vi "sub3.vi"(11 "Terminal in":refnum<vi>) -> (3 "Argument":T1)   [LabVIEW 2020, in "CSM-Helper.lvclass"]
uses:
  CSM-Helper.lvclass
  Typedef/Def-Argument Info.ctl
  <userlib>/_NEVSTOP/Communicable State Machine(CSM)/Communicable State Machine.lvlib
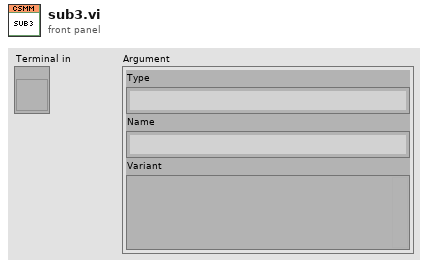
[diagram p1: front panel]
types:
  T1 = typedef "CSM-Helper.lvclass/Def-Argument Info.ctl" = cluster{"Type":string, "Name":string, "Variant":variant}
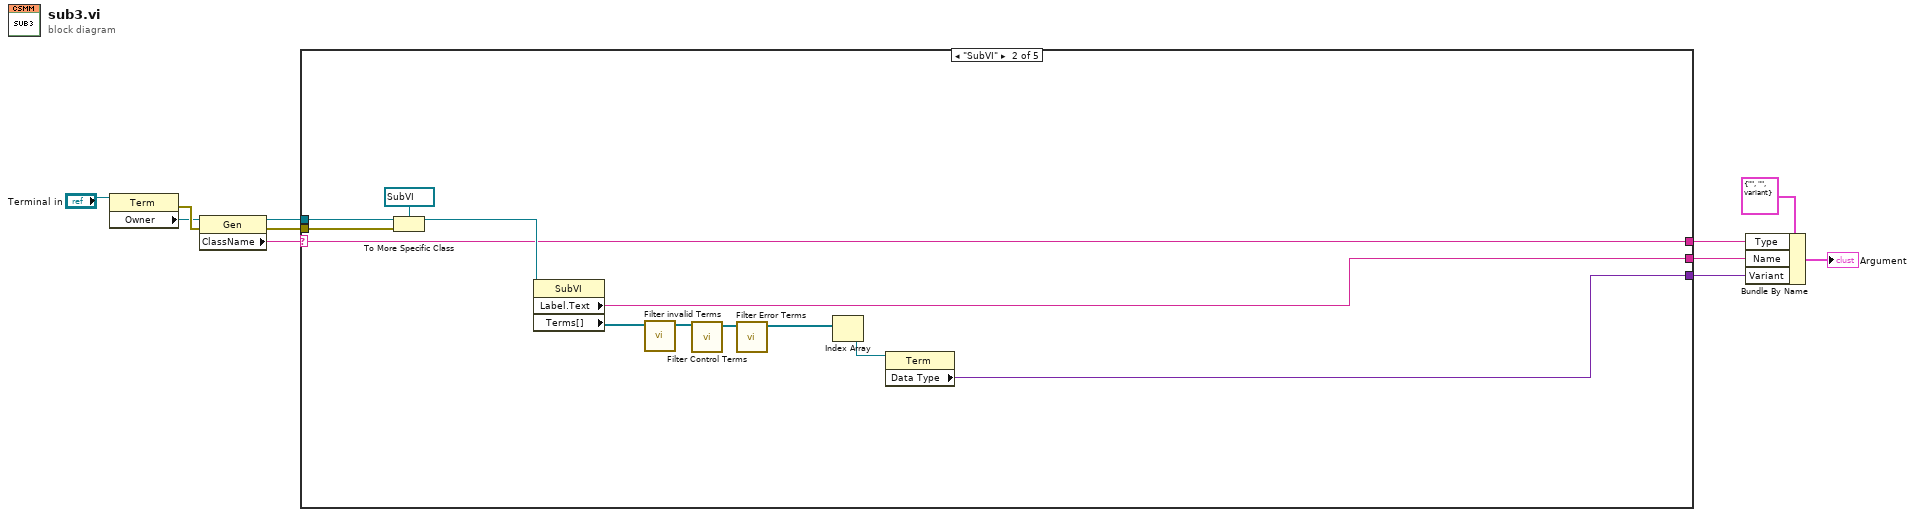
[diagram p0: block diagram]
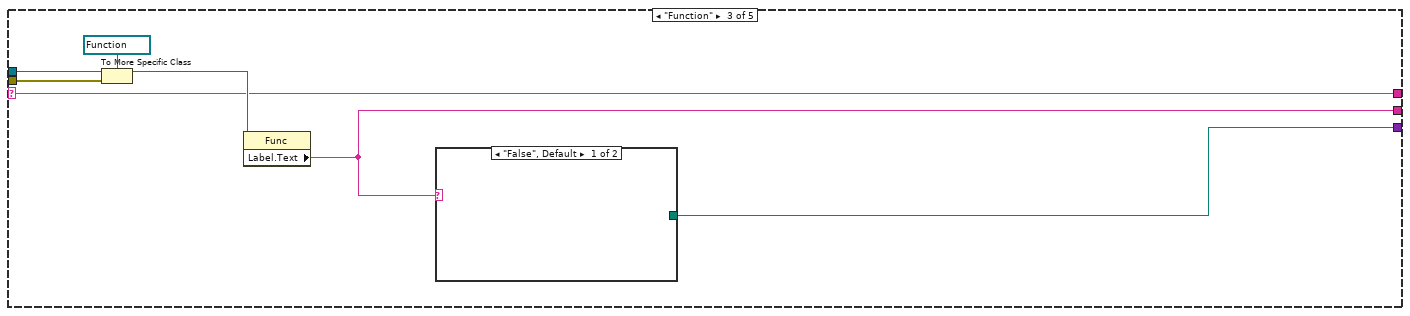
[diagram p3: hidden frame]
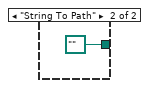
[diagram p4: hidden frame]
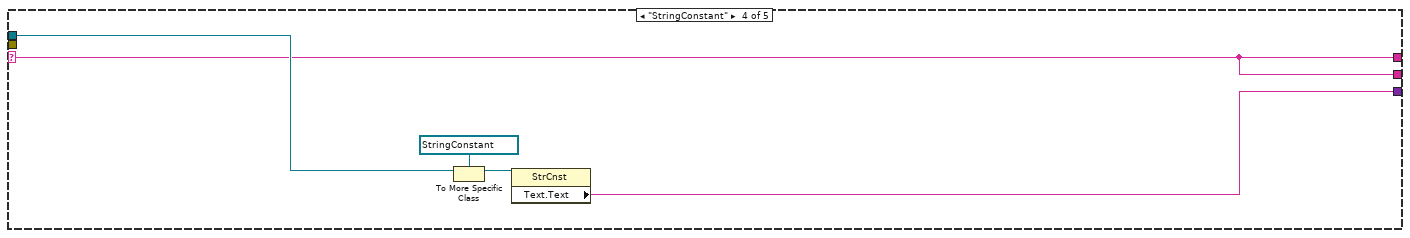
[diagram p5: hidden frame]
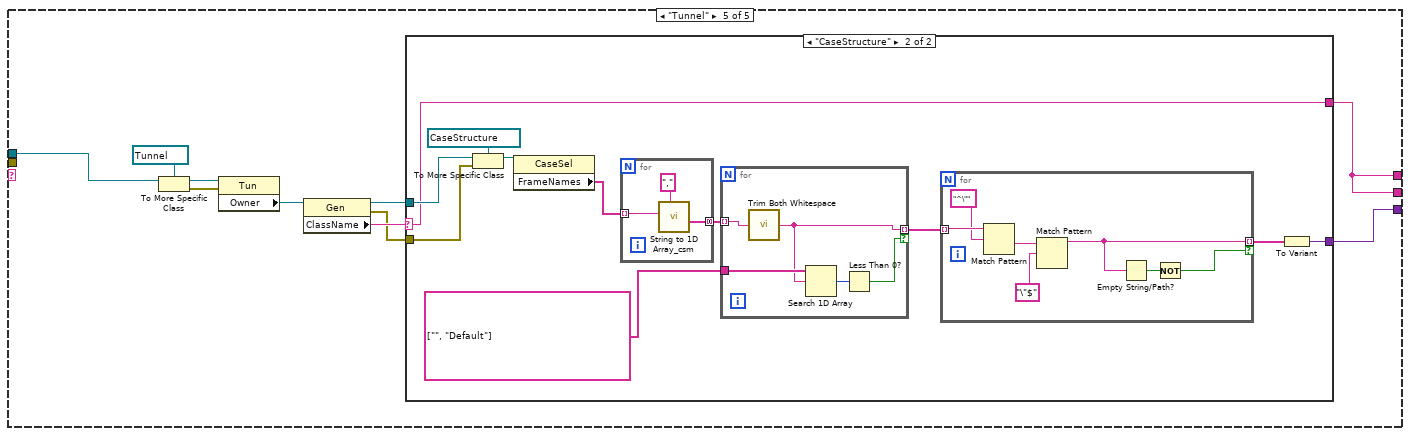
[diagram p6: hidden frame]
diagram:
  n1 = property class="Term"(reference="Terminal in") -> (error out=w6:errorcluster, "Owner"=w4:refnum<vi>)  [unwired: 1 in, 1 out]
  n2 = property class="Gen"(reference=w4, error in=w6) -> (reference out=w5:refnum<vi>, error out=w1:errorcluster, "ClassName"=w8:string)
  n3 = case shown="\"SubVI\"" w8 {
    selector: w8 -> [w12 w20 w28 w33 _]
    tunnel: w5 -> [_ w22 w29 w35 w46]
    tunnel: [_ w21 w26 w33 w38] -> w9
    tunnel: [_ w13 w25 w34 w47] -> w10
    tunnel: [w12 w20 w28 w33 w38] -> w2
    tunnel: w1 -> [_ w19 w27 _ _]
    frame Default {
    }
    frame "SubVI" {
      n4 = To More Specific Class(target class=refnum<vi> refnum ("reference out"), reference=w22, error in=w19) -> (specific class reference=w23:refnum<vi>)  [unwired: 1 out]
      n5 = property class="SubVI"(reference=w23) -> ("Label.Text"=w21:string, "Terms[]"=w16:refnum<vi>[])  [unwired: 1 in, 2 out]
      n6 = call "Filter invalid Terms.vi"("Terms[]"=w16) -> ("Terms[] out"=w17:refnum<vi>[])  [unwired: 10 in]
      n7 = call "Filter Control Terms.vi"("Terms[]"=w17) -> ("Terms[] out"=w18:refnum<vi>[])  [unwired: 10 in]
      n8 = call "Filter Error Terms.vi"("Terms[]"=w18) -> ("Terms[] out"=w15:refnum<vi>[])  [unwired: 10 in]
      n9 = Index Array(array=w15) -> (element=w14:refnum<vi>)  [unwired: 1 in]
      n10 = property class="Term"(reference=w14) -> ("Data Type"=w13:variant)  [unwired: 1 in, 2 out]
    }
    frame "Function" {
      n11 = To More Specific Class(target class=refnum<vi> refnum ("reference out"), reference=w29, error in=w27) -> (specific class reference=w30:refnum<vi>)  [unwired: 1 out]
      n12 = property class="Func"(reference=w30) -> ("Label.Text"=w26:string)  [unwired: 1 in, 2 out]
      n13 = case shown="\"False\", Default" w26 {
        tunnel: [_ path ""] -> w25
        frame "False", Default {
        }
        frame "String To Path" {
        }
      }
    }
    frame "StringConstant" {
      n14 = To More Specific Class(target class=refnum<vi> refnum ("reference out"), reference=w35) -> (specific class reference=w37:refnum<vi>)  [unwired: 1 in, 1 out]
      n15 = property class="StrCnst"(reference=w37) -> ("Text.Text"=w34:string)  [unwired: 1 in, 2 out]
    }
    frame "Tunnel" {
      n16 = To More Specific Class(target class=refnum<vi> refnum ("reference out"), reference=w46) -> (specific class reference=w44:refnum<vi>, error out=w43:errorcluster)  [unwired: 1 in]
      n17 = property class="Tun"(reference=w44, error in=w43) -> ("Owner"=w42:refnum<vi>)  [unwired: 2 out]
      n18 = property class="Gen"(reference=w42) -> (reference out=w40:refnum<vi>, error out=w39:errorcluster, "ClassName"=w41:string)  [unwired: 1 in]
      n19 = case shown="\"CaseStructure\"" w41 {
        selector: w41 -> [w48 w52]
        tunnel: [_ w55] -> w47
        tunnel: w40 -> [_ w54]
        tunnel: w39 -> [_ w53]
        tunnel: [w48 w52] -> w38
        frame Default {
        }
        frame "CaseStructure" {
          n20 = To More Specific Class(target class=refnum<vi> refnum ("reference out"), reference=w54, error in=w53) -> (specific class reference=w59:refnum<vi>)  [unwired: 1 out]
          n21 = property class="CaseSel"(reference=w59) -> ("FrameNames"=w56:string[])  [unwired: 1 in, 2 out]
          n22 = for {
            tunnel: [w66] -> w57 mode=concatenating
            tunnel: w56 -> [w65] mode=indexing
            n23 = call <userlib>:"String to 1D Array_csm.vi"("delimiter (Tab)"=",", "string"=w65) -> ("Array of Strings"=w66:string[])  [unwired: 9 in]
          }
          n24 = for {
            tunnel: [w62] -> w49 mode=indexing if=w60
            tunnel: w57 -> [w64] mode=indexing
            tunnel: string[] ["", "Default"] ("items to filter") -> [w63]
            n25 = call <userlib>:"Trim Both Whitespace.vi"("string"=w64) -> ("trimmed string"=w62:string)  [unwired: 1 in]
            n26 = Search 1D Array(1D array=w63, element=w62) -> (index of element=w61:i32)  [unwired: 1 in]
            n27 = Less Than 0?(x=w61) -> (x < 0?=w60:bool)
          }
          n28 = for {
            tunnel: w49 -> [w74] mode=indexing
            tunnel: [w70] -> w51 mode=indexing if=w69
            n29 = Match Pattern(string=w74, regular expression="^\"") -> (after substring=w72:string)  [unwired: 1 in, 3 out]
            n30 = Match Pattern(string=w72, regular expression="\"$") -> (before substring=w70:string)  [unwired: 1 in, 3 out]
            n31 = Empty String/Path?(string/path=w70) -> (empty?=w68:bool)
            n32 = Not(x=w68) -> (.not. x?=w69:bool)
          }
          n33 = To Variant(anything=w51) -> (Variant=w55:variant)
        }
      }
    }
  }
  n34 = Bundle By Name(cluster=T1 {"Type"="", "Name"="", "Variant"=variant} ("Argument"), "Type"=w2, "Name"=w9, "Variant"=w10) -> (→"Argument":T1)
